vi "TrajectoryParam_enforceAccel.vi"(8 "TRAJECTORY_CONFIG":T1={"MaxVelocity"=0.0, "Max Acceleration"=0.0, "StartVelocity"=0.0, "End Velocity"=0.0, "Reversed"=FALSE, "DiffDrKineConstntDefined"=FALSE, "CentAcellConstntDefined"=FALSE, "DiffDrVoltConstntDefined"=FALSE, "DIFF_DRIVE_KINE_CONSTRAINT"={"Max Speed (M/S)"=0.0, "DIFF_DRIVE_KINEMATICS"={"TrackWidth_Meters"=0.0}}, "CENTRIPETAL_ACCEL_CONSTRAINT"={"Max Cent Accel"=0.0}, "SwerveDrKineConstntDefined"=FALSE, "SWERVE_DRIVE_KINE_CONSTRAINT"={"Max Speed (M/S)"=0.0, "SwerveKinematics"={"NumModules"=0, "InverseKinematics"=[], "ForwardKinematics"=[], "Modules"=[], "PrevCoR"={"X"=0.0, "Y"=0.0}}}, "DIFF_DRIVE_VOLTAGE_CONSTRAINT"={"Max Voltage"=0.0, "DIFF_DRIVE_KINEMATICS"={"TrackWidth_Meters"=0.0}, "SIMPLE_MOTOR_FF"={"Ks"=0.0, "Kv"=0.0, "Ka"=0.0}}, "MECANUM_DRIVE_KINE_CONSTRAINT"={"Max Speed (M/S)"=0.0, "MECA_DRIVE_KINEMATICS"={"FrontLeft"={"X"=0.0, "Y"=0.0}, "FrontRight"={"X"=0.0, "Y"=0.0}, "RearLeft"={"X"=0.0, "Y"=0.0}, "RearRight"={"X"=0.0, "Y"=0.0}, "InverseKinematics"=[[0.0, 1.0, -1.0, 0.0], [0.0, 1.0, 1.0, 0.0], [0.0, 1.0, 1.0, 0.0], [0.0, 1.0, -1.0, 0.0]], "ForwardKinematics"=[[0.0, 1.0, -1.0, 0.0], [0.0, 1.0, 1.0, 0.0], [0.0, 1.0, 1.0, 0.0], [0.0, 1.0, -1.0, 0.0]], "PrevCoR"={"X"=0.0, "Y"=0.0}}}, "MecanumDrKineConstntDefined"=FALSE} {"MECANUM_DRIVE_KINE_CONSTRAINT"."MECA_DRIVE_KINEMATICS"."PrevCoR"."Y" format="%14.3f"; "MECANUM_DRIVE_KINE_CONSTRAINT"."MECA_DRIVE_KINEMATICS"."PrevCoR"."X" format="%14.3f"; "MECANUM_DRIVE_KINE_CONSTRAINT"."MECA_DRIVE_KINEMATICS"."RearRight"."Y" format="%14.3f"; "MECANUM_DRIVE_KINE_CONSTRAINT"."MECA_DRIVE_KINEMATICS"."RearRight"."X" format="%14.3f"; "MECANUM_DRIVE_KINE_CONSTRAINT"."MECA_DRIVE_KINEMATICS"."RearLeft"."Y" format="%14.3f"; "MECANUM_DRIVE_KINE_CONSTRAINT"."MECA_DRIVE_KINEMATICS"."RearLeft"."X" format="%14.3f"; "MECANUM_DRIVE_KINE_CONSTRAINT"."MECA_DRIVE_KINEMATICS"."FrontRight"."Y" format="%14.3f"; "MECANUM_DRIVE_KINE_CONSTRAINT"."MECA_DRIVE_KINEMATICS"."FrontRight"."X" format="%14.3f"; "MECANUM_DRIVE_KINE_CONSTRAINT"."MECA_DRIVE_KINEMATICS"."FrontLeft"."Y" format="%14.3f"; "MECANUM_DRIVE_KINE_CONSTRAINT"."MECA_DRIVE_KINEMATICS"."FrontLeft"."X" format="%14.3f"; "MECANUM_DRIVE_KINE_CONSTRAINT"."Max Speed (M/S)" format="%20.4f"; "DIFF_DRIVE_VOLTAGE_CONSTRAINT"."SIMPLE_MOTOR_FF"."Ka" format="%13.4f"; "DIFF_DRIVE_VOLTAGE_CONSTRAINT"."SIMPLE_MOTOR_FF"."Kv" format="%13.4f"; "DIFF_DRIVE_VOLTAGE_CONSTRAINT"."SIMPLE_MOTOR_FF"."Ks" format="%13.4f"; "DIFF_DRIVE_VOLTAGE_CONSTRAINT"."DIFF_DRIVE_KINEMATICS"."TrackWidth_Meters" format="%20.4f"; "DIFF_DRIVE_VOLTAGE_CONSTRAINT"."Max Voltage" format="%20.4f"; "SWERVE_DRIVE_KINE_CONSTRAINT"."SwerveKinematics"."PrevCoR"."Y" format="%14.3f"; "SWERVE_DRIVE_KINE_CONSTRAINT"."SwerveKinematics"."PrevCoR"."X" format="%14.3f"; "SWERVE_DRIVE_KINE_CONSTRAINT"."SwerveKinematics"."Modules"."Y" format="%14.3f"; "SWERVE_DRIVE_KINE_CONSTRAINT"."SwerveKinematics"."Modules"."X" format="%14.3f"; "SWERVE_DRIVE_KINE_CONSTRAINT"."Max Speed (M/S)" format="%20.4f"; "CENTRIPETAL_ACCEL_CONSTRAINT"."Max Cent Accel" format="%20.4f"; "DIFF_DRIVE_KINE_CONSTRAINT"."DIFF_DRIVE_KINEMATICS"."TrackWidth_Meters" format="%20.4f"; "DIFF_DRIVE_KINE_CONSTRAINT"."Max Speed (M/S)" format="%20.4f"; "End Velocity" format="%20.4f"; "StartVelocity" format="%20.4f"; "Max Acceleration" format="%20.4f"; "MaxVelocity" format="%20.4f"}, 10 "Reversed":bool, 11 "inCONSTRAINED_STATE":T13={"POSEwCURVATURE"={"CURVATURE"=0.0, "POSE"={"TRANSLATION"={"X"=0.0, "Y"=0.0}, "ROTATION"={"VALUE"=0.0, "COS"=1.0, "SIN"=0.0}}}, "Distance"=0.0, "minAccel"=0.0, "maxAccel"=0.0, "maxVelocity"=0.0} {"POSEwCURVATURE"."POSE"."ROTATION"."SIN" format="%13.4f"; "POSEwCURVATURE"."POSE"."ROTATION"."COS" format="%13.4f"; "POSEwCURVATURE"."POSE"."ROTATION"."VALUE" format="%13.4f"; "POSEwCURVATURE"."POSE"."TRANSLATION"."Y" format="%14.3f"; "POSEwCURVATURE"."POSE"."TRANSLATION"."X" format="%14.3f"}) -> (0 "error out":errorcluster, 3 "outCONSTRAINED_STATE":T13={"POSEwCURVATURE"={"CURVATURE"=0.0, "POSE"={"TRANSLATION"={"X"=0.0, "Y"=0.0}, "ROTATION"={"VALUE"=0.0, "COS"=1.0, "SIN"=0.0}}}, "Distance"=0.0, "minAccel"=0.0, "maxAccel"=0.0, "maxVelocity"=0.0} {"POSEwCURVATURE"."POSE"."ROTATION"."SIN" format="%13.4f"; "POSEwCURVATURE"."POSE"."ROTATION"."COS" format="%13.4f"; "POSEwCURVATURE"."POSE"."ROTATION"."VALUE" format="%13.4f"; "POSEwCURVATURE"."POSE"."TRANSLATION"."Y" format="%14.3f"; "POSEwCURVATURE"."POSE"."TRANSLATION"."X" format="%14.3f"})   [LabVIEW 2019, in "Trajectory_Library.lvlib"]
doc: "Internal routine called by TrajectoryParam_timeParam.VI \n\nThis routine enforces acceleration constraints and updates the ConstrainedState value based on the calculated limits.\n\nThis routine will need to be updated whenever a new constrained state type is added.\n------------------------------------------------------------------------------------------\n\nParameters:\n - InConstrainedState\n - Reversed\n - TrajectoryConfig\n\nReturns\n - OutConstrainedState"
uses:
  Trajectory_Library.lvlib
  CONSTRAINED_STATE.ctl
  POSEwCURVATURE.ctl
  POSE2D.ctl
  TRANSLATION2D.ctl
  ROTATION2D.ctl
  TRAJ_CONFIG.ctl
  TRAJ_CONSTRAINT_DIIF_DRIVE_KINEMATICS.ctl
  DIFF_DRIVE_KINEMATICS.ctl
  TRAJ_CONSTRAINT_CENTRIPETAL_ACCEL.ctl
  TRAJ_CONSTRAINT_SWERVE_DRIVE_KINEMATICS.ctl
  SWERVE_DRIVE_KINEMATICS.ctl
  <vilib>/Analysis/Matrix/Datatypes/RealMatrix.ctl
  TRAJ_CONSTRAINT_DIIF_DRIVE_VOLTAGE.ctl
  SIMPLE_MOTOR_FF.ctl
  TRAJ_CONSTRAINT_MECA_DRIVE_KINEMATICS.ctl
  MECA_DRIVE_KINEMATICS.ctl
  <vilib>/Analysis/Matrix/NI_Matrix.lvlib
panel:
  # "ARRAY OF OTHER\nCONSTRAINTS \nGOES HERE.."
  # "All units\nare SI"
  # "All units\nare SI"
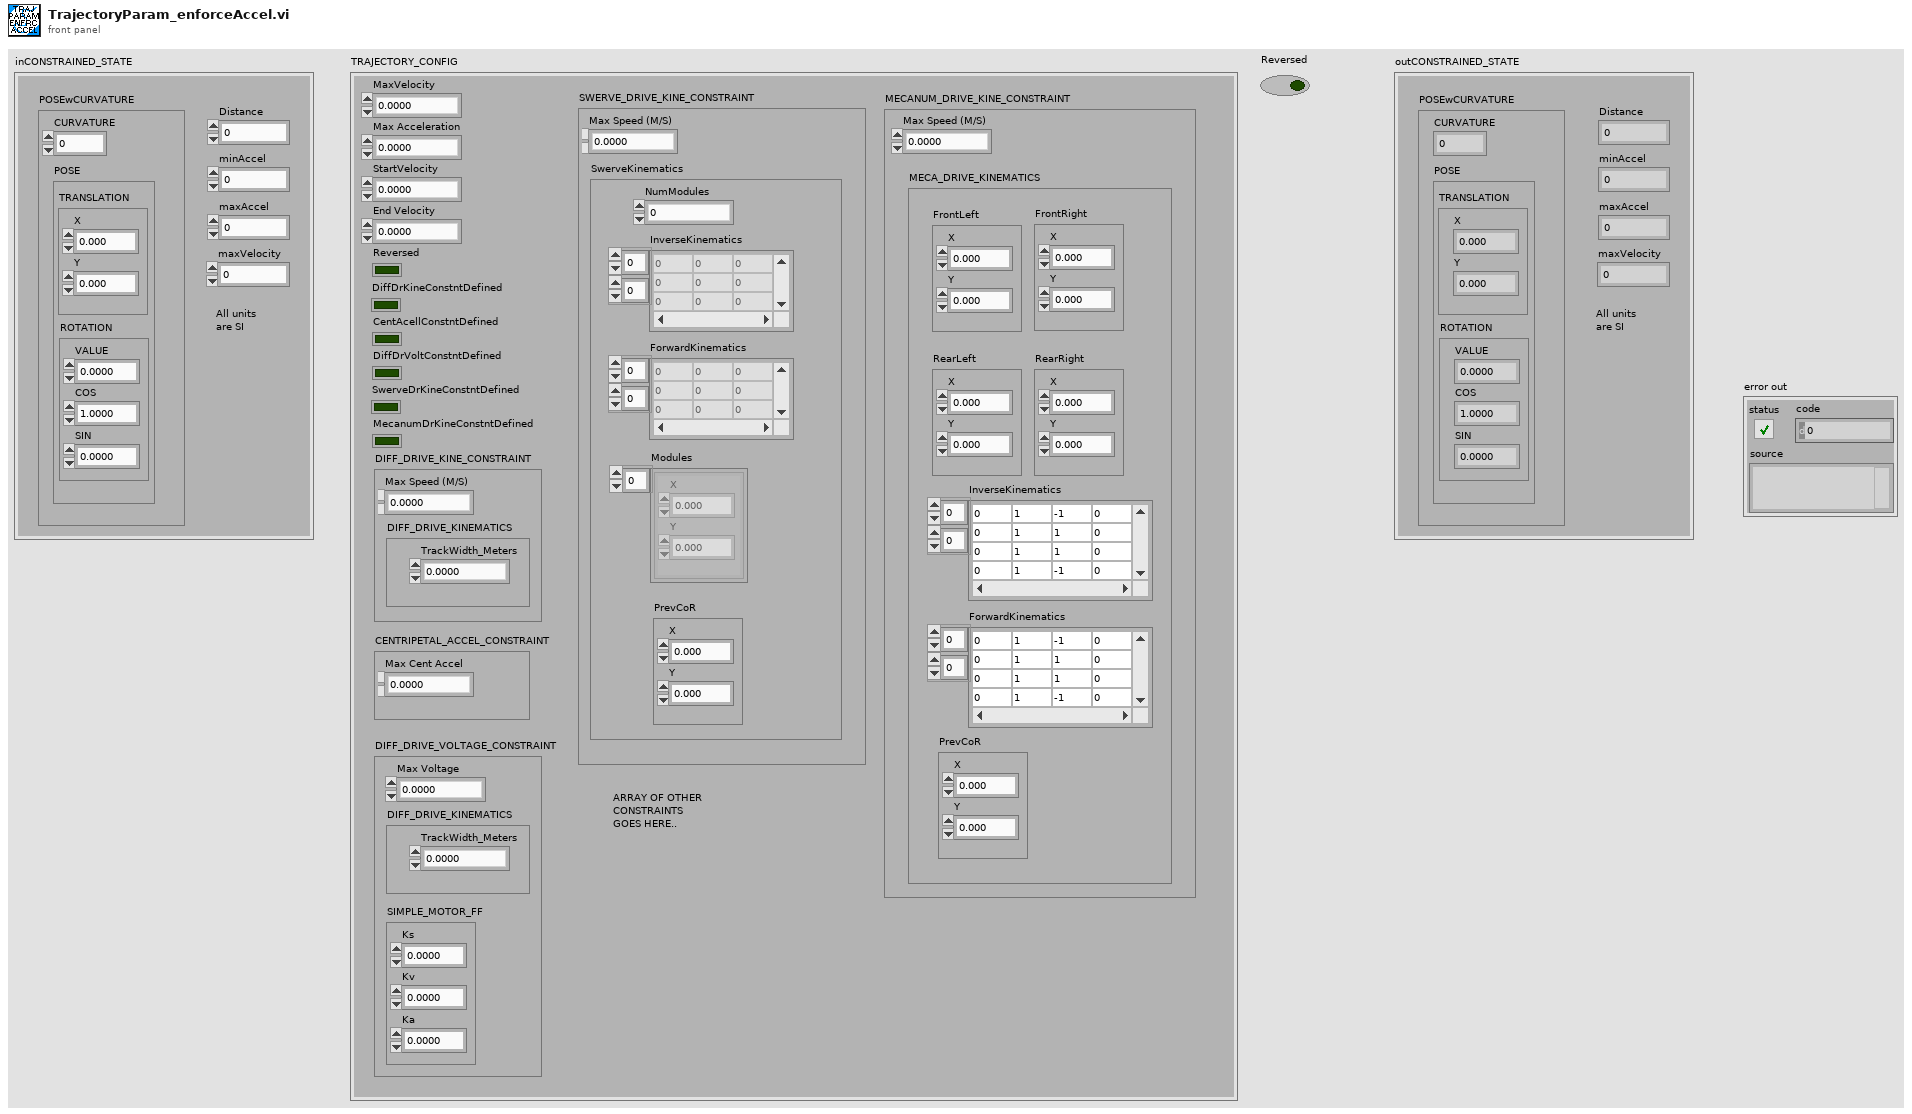
[diagram p1: front panel]
types:
  T1 = typedef "Trajectory_Library.lvlib/TRAJ_CONFIG.ctl" = cluster{"MaxVelocity":dbl, "Max Acceleration":dbl, "StartVelocity":dbl, "End Velocity":dbl, "Reversed":bool, "DiffDrKineConstntDefined":bool, "CentAcellConstntDefined":bool, "DiffDrVoltConstntDefined":bool, "DIFF_DRIVE_KINE_CONSTRAINT":T2, "CENTRIPETAL_ACCEL_CONSTRAINT":T4, "SwerveDrKineConstntDefined":bool, "SWERVE_DRIVE_KINE_CONSTRAINT":T5, "DIFF_DRIVE_VOLTAGE_CONSTRAINT":T9, "MECANUM_DRIVE_KINE_CONSTRAINT":T11, "MecanumDrKineConstntDefined":bool}
  T2 = typedef "Trajectory_Library.lvlib/TRAJ_CONSTRAINT_DIIF_DRIVE_KINEMATICS.ctl" = cluster{"Max Speed (M/S)":dbl, "DIFF_DRIVE_KINEMATICS":T3}
  T3 = typedef "Trajectory_Library.lvlib/DIFF_DRIVE_KINEMATICS.ctl" = cluster{"TrackWidth_Meters":dbl}
  T4 = typedef "Trajectory_Library.lvlib/TRAJ_CONSTRAINT_CENTRIPETAL_ACCEL.ctl" = cluster{"Max Cent Accel":dbl}
  T5 = typedef "Trajectory_Library.lvlib/TRAJ_CONSTRAINT_SWERVE_DRIVE_KINEMATICS.ctl" = cluster{"Max Speed (M/S)":dbl, "SwerveKinematics":T6}
  T6 = typedef "Trajectory_Library.lvlib/SWERVE_DRIVE_KINEMATICS.ctl" = cluster{"NumModules":i32, "InverseKinematics":T7, "ForwardKinematics":T7, "Modules":T8[], "PrevCoR":T8}
  T7 = typedef "NI_Matrix.lvlib/RealMatrix.ctl" = dbl[][]
  T8 = typedef "Trajectory_Library.lvlib/TRANSLATION2D.ctl" = cluster{"X":dbl, "Y":dbl}
  T9 = typedef "Trajectory_Library.lvlib/TRAJ_CONSTRAINT_DIIF_DRIVE_VOLTAGE.ctl" = cluster{"Max Voltage":dbl, "DIFF_DRIVE_KINEMATICS":T3, "SIMPLE_MOTOR_FF":T10}
  T10 = typedef "Trajectory_Library.lvlib/SIMPLE_MOTOR_FF.ctl" = cluster{"Ks":dbl, "Kv":dbl, "Ka":dbl}
  T11 = typedef "Trajectory_Library.lvlib/TRAJ_CONSTRAINT_MECA_DRIVE_KINEMATICS.ctl" = cluster{"Max Speed (M/S)":dbl, "MECA_DRIVE_KINEMATICS":T12}
  T12 = typedef "Trajectory_Library.lvlib/MECA_DRIVE_KINEMATICS.ctl" = cluster{"FrontLeft":T8, "FrontRight":T8, "RearLeft":T8, "RearRight":T8, "InverseKinematics":T7, "ForwardKinematics":T7, "PrevCoR":T8}
  T13 = typedef "Trajectory_Library.lvlib/CONSTRAINED_STATE.ctl" = cluster{"POSEwCURVATURE":T14, "Distance":dbl, "minAccel":dbl, "maxAccel":dbl, "maxVelocity":dbl}
  T14 = typedef "Trajectory_Library.lvlib/POSEwCURVATURE.ctl" = cluster{"CURVATURE":dbl, "POSE":T15}
  T15 = typedef "Trajectory_Library.lvlib/POSE2D.ctl" = cluster{"TRANSLATION":T8, "ROTATION":T16}
  T16 = typedef "Trajectory_Library.lvlib/ROTATION2D.ctl" = cluster{"VALUE":dbl, "COS":dbl, "SIN":dbl}
  T17 = typedef "Trajectory_Library.lvlib/TRAJ_CONSTRAINT_MINMAX.ctl" = cluster{"minAccel":dbl, "maxAccel":dbl}
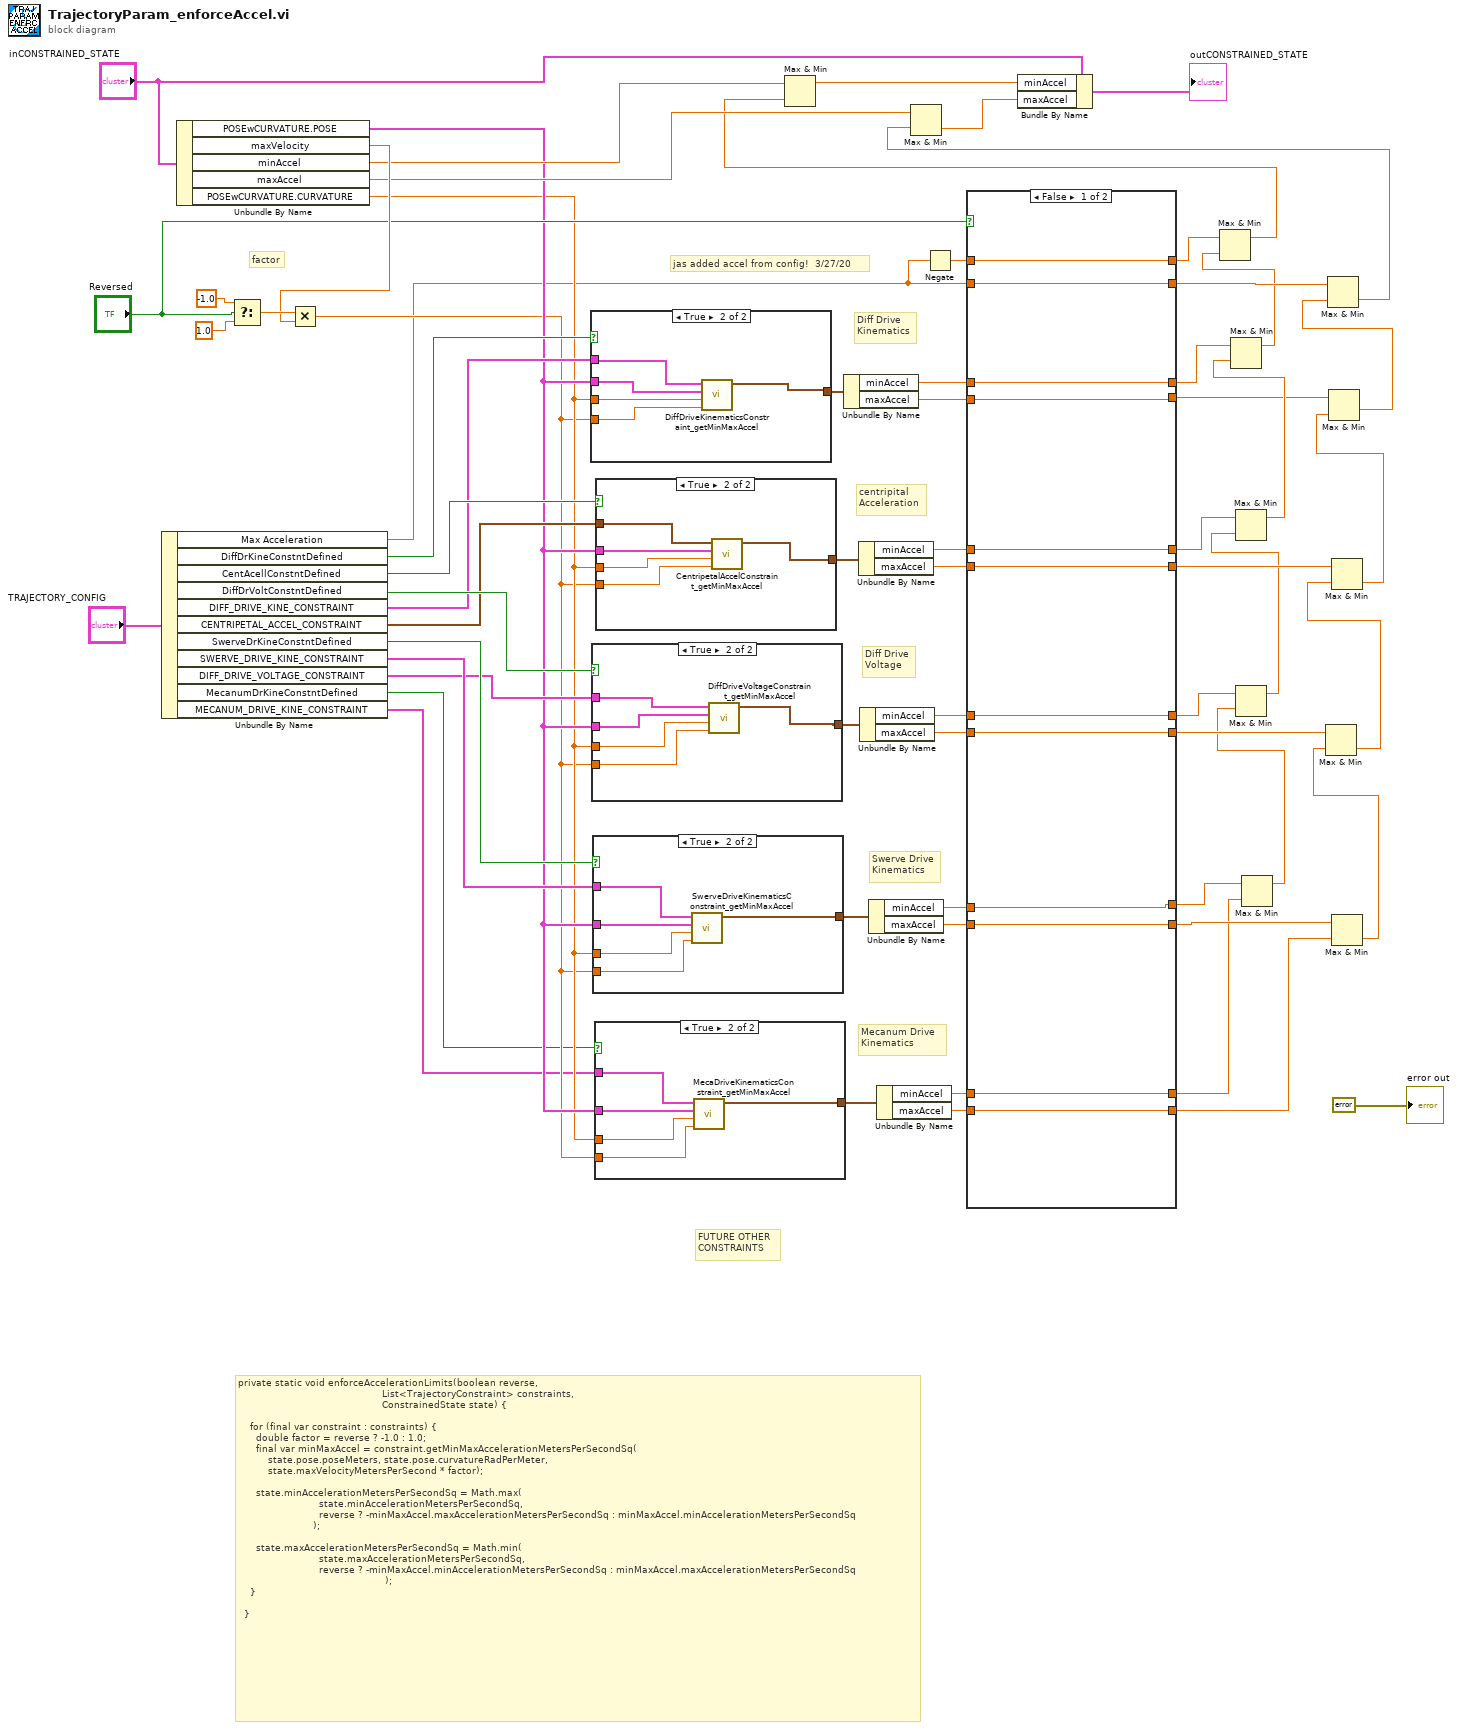
[diagram p0: block diagram]
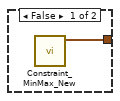
[diagram p2: hidden frame]
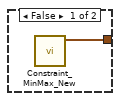
[diagram p3: hidden frame]
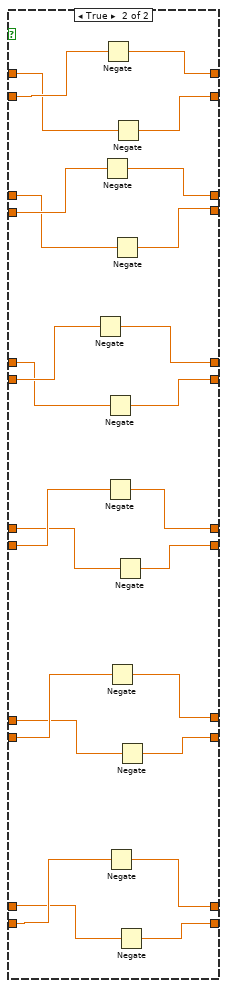
[diagram p4: hidden frame]
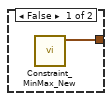
[diagram p5: hidden frame]
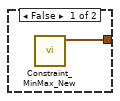
[diagram p6: hidden frame]
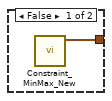
[diagram p7: hidden frame]
diagram:
  # "jas added accel from config!  3/27/20"
  # "Mecanum Drive\nKinematics"
  # "Swerve Drive\nKinematics"
  # "factor"
  # "Diff Drive\nVoltage"
  # "centripital\nAcceleration"
  # "Diff Drive \nKinematics"
  # "FUTURE OTHER\nCONSTRAINTS"
  # "private static void enforceAccelerationLimits(boolean reverse,\n                                                List<TrajectoryConstraint> constraints,\n                                                ConstrainedState state) {\n\n    for (final var constraint : constraints) {\n      double factor = reverse ? -1.0 : 1.0;\n      final var minMaxAccel = constraint.getMinMaxAccelerationMetersPerSecondSq(\n          state.pose.poseMeters, state.pose.curvatureRadPerMeter,\n          state.maxVelocityMetersPerSecond * factor);\n\n      state.minAccelerationMetersPerSecondSq = Math.max(\n                           state.minAccelerationMetersPerSecondSq,\n                           reverse ? -minMaxAccel.maxAccelerationMetersPerSecondSq : minMaxAccel.minAccelerationMetersPerSecondSq\n                         );\n\n      state.maxAccelerationMetersPerSecondSq = Math.min(\n                           state.maxAccelerationMetersPerSecondSq,\n                           reverse ? -minMaxAccel.minAccelerationMetersPerSecondSq : minMaxAccel.maxAccelerationMetersPerSecondSq\n                                                 );\n    }\n\n  }"
  n1 = Unbundle By Name("TRAJECTORY_CONFIG") -> ("Max Acceleration"=w3:dbl, "DiffDrKineConstntDefined"=w61:bool, "CentAcellConstntDefined"=w60:bool, "DiffDrVoltConstntDefined"=w59:bool, "DIFF_DRIVE_KINE_CONSTRAINT"=w58:T2, "CENTRIPETAL_ACCEL_CONSTRAINT"=w33:T4, "SwerveDrKineConstntDefined"=w29:bool, "SWERVE_DRIVE_KINE_CONSTRAINT"=w28:T5, "DIFF_DRIVE_VOLTAGE_CONSTRAINT"=w23:T9, "MecanumDrKineConstntDefined"=w10:bool, "MECANUM_DRIVE_KINE_CONSTRAINT"=w9:T11)
  n2 = Unbundle By Name("inCONSTRAINED_STATE") -> ("POSEwCURVATURE.POSE"=w22:T15, "maxVelocity"=w56:dbl, "minAccel"=w42:dbl, "maxAccel"=w34:dbl, "POSEwCURVATURE.CURVATURE"=w21:dbl)
  n3 = Select(t=-1.0, s="Reversed", f=1.0) -> (s? t:f=w57:dbl)
  n4 = Multiply(x=w57, y=w56) -> (x*y=w20:dbl)
  n5 = case shown="True" w61 {
    tunnel: [w66 w71] -> w53
    tunnel: w58 -> [_ w70]
    tunnel: w22 -> [_ w69]
    tunnel: w20 -> [_ w67]
    tunnel: w21 -> [_ w68]
    frame False {
      n6 = call "Constraint_MinMax_New.vi"() -> ("TRAJ_CONSTAINT_MIN_MAX"=w66:T17)  [unwired: 11 in]
    }
    frame True {
      n7 = call "DiffDriveKinematicsConstraint_getMinMaxAccel.vi"("maxVelocity"=w67, "Curvature"=w68, "statePose"=w69, "DIFF_DRIVE_KINE_CONSTRAINT"=w70) -> ("TRAJ_CONSTAINT_MIN_MAX"=w71:T17)  [unwired: 7 in]
    }
  }
  n8 = case shown="True" w59 {
    tunnel: [w72 w77] -> w51
    tunnel: w22 -> [_ w75]
    tunnel: w20 -> [_ w73]
    tunnel: w21 -> [_ w74]
    tunnel: w23 -> [_ w76]
    frame False {
      n9 = call "Constraint_MinMax_New.vi"() -> ("TRAJ_CONSTAINT_MIN_MAX"=w72:T17)  [unwired: 11 in]
    }
    frame True {
      n10 = call "DiffDriveVoltageConstraint_getMinMaxAccel.vi"("Velocity"=w73, "Curvature"=w74, "statePose"=w75, "DIFF_DRIVE_VOLTAGE_CONSTRAINT"=w76) -> ("TRAJ_CONSTAINT_MIN_MAX"=w77:T17)  [unwired: 7 in]
    }
  }
  n11 = case shown="True" w29 {
    tunnel: [w78 w83] -> w30
    tunnel: w21 -> [_ w82]
    tunnel: w20 -> [_ w81]
    tunnel: w22 -> [_ w80]
    tunnel: w28 -> [_ w79]
    frame False {
      n12 = call "Constraint_MinMax_New.vi"() -> ("TRAJ_CONSTAINT_MIN_MAX"=w78:T17)  [unwired: 11 in]
    }
    frame True {
      n13 = call "SwerveDriveKinematicsConstraint_getMinMaxAccel.vi"("maxVelocity"=w81, "Curvature"=w82, "statePose"=w80, "SWERVE_DRIVE_KINE_CONSTRAINT"=w79) -> ("TRAJ_CONSTAINT_MIN_MAX"=w83:T17)  [unwired: 7 in]
    }
  }
  n14 = case shown="True" w10 {
    tunnel: [w84 w89] -> w19
    tunnel: w21 -> [_ w88]
    tunnel: w20 -> [_ w87]
    tunnel: w22 -> [_ w86]
    tunnel: w9 -> [_ w85]
    frame False {
      n15 = call "Constraint_MinMax_New.vi"() -> ("TRAJ_CONSTAINT_MIN_MAX"=w84:T17)  [unwired: 11 in]
    }
    frame True {
      n16 = call "MecaDriveKinematicsConstraint_getMinMaxAccel.vi"("maxVelocity"=w87, "Curvature"=w88, "statePose"=w86, "MECANUM_DRIVE_KINE_CONSTRAINT"=w85) -> ("TRAJ_CONSTAINT_MIN_MAX"=w89:T17)  [unwired: 7 in]
    }
  }
  n17 = case shown="True" w60 {
    tunnel: [w90 w91] -> w52
    tunnel: w22 -> [_ w94]
    tunnel: w20 -> [_ w92]
    tunnel: w33 -> [_ w95]
    tunnel: w21 -> [_ w93]
    frame False {
      n18 = call "Constraint_MinMax_New.vi"() -> ("TRAJ_CONSTAINT_MIN_MAX"=w90:T17)  [unwired: 11 in]
    }
    frame True {
      n19 = call "CentripetalAccelConstraint_getMinMaxAccel.vi"("maxVelocity"=w92, "Curvature"=w93, "statePose"=w94, "CENTRIPETAL_ACCEL_CONSTRAINT"=w95) -> ("TRAJ_CONSTAINT_MIN_MAX"=w91:T17)  [unwired: 7 in]
    }
  }
  n20 = Unbundle By Name(w53) -> ("minAccel"=w49:dbl, "maxAccel"=w48:dbl)
  n21 = Unbundle By Name(w52) -> ("minAccel"=w47:dbl, "maxAccel"=w46:dbl)
  n22 = Unbundle By Name(w51) -> ("minAccel"=w45:dbl, "maxAccel"=w44:dbl)
  n23 = Unbundle By Name(w30) -> ("minAccel"=w31:dbl, "maxAccel"=w32:dbl)
  n24 = Unbundle By Name(w19) -> ("minAccel"=w18:dbl, "maxAccel"=w17:dbl)
  n25 = Negate(x=w3) -> (-x=w2:dbl)
  n26 = case shown="False" "Reversed" {
    tunnel: [w107 w130] -> w40
    tunnel: w49 -> [w107 w125]
    tunnel: [w106 w124] -> w36
    tunnel: w48 -> [w106 w131]
    tunnel: [w105 w128] -> w43
    tunnel: w47 -> [w105 w123]
    tunnel: [w104 w122] -> w38
    tunnel: w46 -> [w104 w129]
    tunnel: [w103 w126] -> w27
    tunnel: w45 -> [w103 w121]
    tunnel: [w102 w120] -> w25
    tunnel: w44 -> [w102 w127]
    tunnel: w32 -> [w100 w119]
    tunnel: w31 -> [w101 w118]
    tunnel: [w101 w117] -> w15
    tunnel: [w100 w116] -> w16
    tunnel: w18 -> [w99 w114]
    tunnel: w17 -> [w98 w115]
    tunnel: [w99 w113] -> w12
    tunnel: [w98 w112] -> w11
    tunnel: w3 -> [w97 w109]
    tunnel: [w97 w110] -> w8
    tunnel: w2 -> [w96 w108]
    tunnel: [w96 w111] -> w1
    frame False {
    }
    frame True {
      n27 = Negate(x=w129) -> (-x=w128:dbl)
      n28 = Negate(x=w131) -> (-x=w130:dbl)
      n29 = Negate(x=w109) -> (-x=w111:dbl)
      n30 = Negate(x=w123) -> (-x=w122:dbl)
      n31 = Negate(x=w127) -> (-x=w126:dbl)
      n32 = Negate(x=w115) -> (-x=w113:dbl)
      n33 = Negate(x=w119) -> (-x=w117:dbl)
      n34 = Negate(x=w125) -> (-x=w124:dbl)
      n35 = Negate(x=w108) -> (-x=w110:dbl)
      n36 = Negate(x=w121) -> (-x=w120:dbl)
      n37 = Negate(x=w114) -> (-x=w112:dbl)
      n38 = Negate(x=w118) -> (-x=w116:dbl)
    }
  }
  n39 = Max & Min(x=w15, y=w12) -> (max(x,y)=w14:dbl)  [unwired: 1 out]
  n40 = Max & Min(x=w27, y=w14) -> (max(x,y)=w26:dbl)  [unwired: 1 out]
  n41 = Max & Min(x=w43, y=w26) -> (max(x,y)=w39:dbl)  [unwired: 1 out]
  n42 = Max & Min(x=w40, y=w39) -> (max(x,y)=w4:dbl)  [unwired: 1 out]
  n43 = Max & Min(x=w1, y=w4) -> (max(x,y)=w5:dbl)  [unwired: 1 out]
  n44 = Max & Min(x=w42, y=w5) -> (max(x,y)=w41:dbl)  [unwired: 1 out]
  n45 = Max & Min(x=w16, y=w11) -> (min(x,y)=w13:dbl)  [unwired: 1 out]
  n46 = Max & Min(x=w25, y=w13) -> (min(x,y)=w24:dbl)  [unwired: 1 out]
  n47 = Max & Min(x=w38, y=w24) -> (min(x,y)=w37:dbl)  [unwired: 1 out]
  n48 = Max & Min(x=w36, y=w37) -> (min(x,y)=w6:dbl)  [unwired: 1 out]
  n49 = Max & Min(x=w8, y=w6) -> (min(x,y)=w7:dbl)  [unwired: 1 out]
  n50 = Max & Min(x=w34, y=w7) -> (min(x,y)=w35:dbl)  [unwired: 1 out]
  n51 = Bundle By Name(cluster="inCONSTRAINED_STATE", "minAccel"=w41, "maxAccel"=w35) -> (→"outCONSTRAINED_STATE":T13)
  "error out" <- errorcluster {"status"=FALSE, "code"=0, "source"=""} ("error out")
